vi "PLL Final.vi"() -> ()   [LabVIEW 2009]
uses:
  <vilib>/Instr/_visa.llb/VISA Configure Serial Port (Instr).vi
panel:
  in  "SDR RS232 CONTROLLER 2":T1(tab)
  in  "Stop":bool
  in  "Verzend":bool
  in  "BAND SELECTOR":dbl(ring)
  out "Ingesteld?":bool
  in  "VISA resource name":refnum<visa-resource-name>="COM1"
  in  "data bits":u16=8 min=5 max=8 step=1
  in  "baud rate":u32=9600
  out "Ingestelde frequenties":dbl(graph)
  # "PRIORITY SETTINGS"
  # "Software Defined Radio Controller SDRC3264 English\n\n  Copyright (C) 2010-2011 , All rights reserved.\n  \n\n  Software Defined Radio is being developed by:\n                - Jeroen Croes\n                - Elisa Staelen\n                - Tom Grenson\n\n\n\n  This software is packaged using NI LabView by National Instruments\n  (www.http://www.ni.com/labview/)."
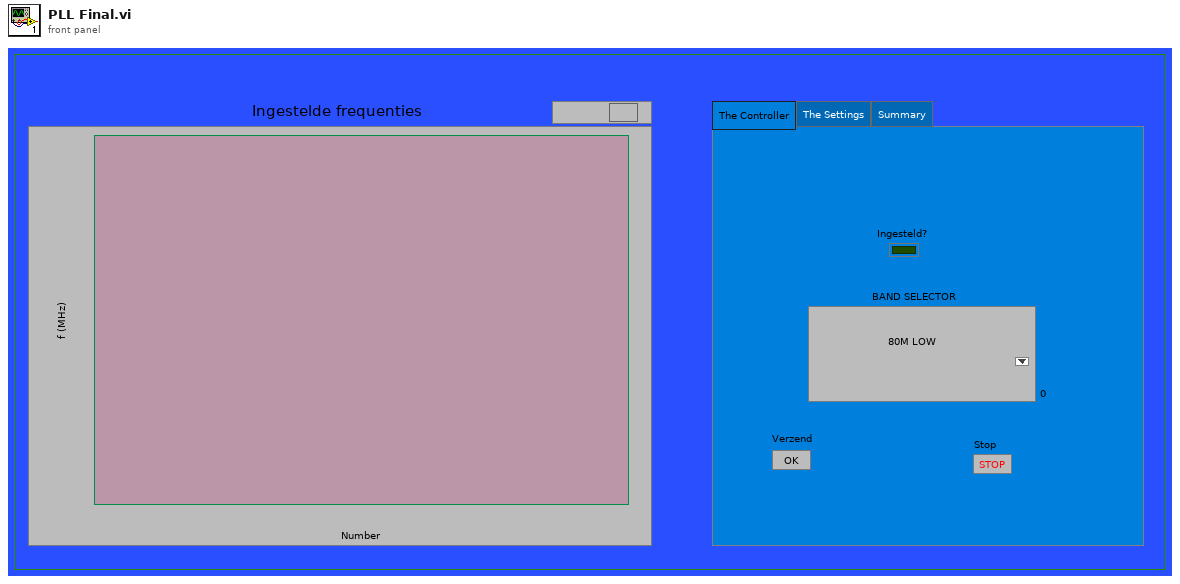
[diagram p1: front panel]
types:
  T1 = enum32{"The Controller", "The Settings", "Summary"}
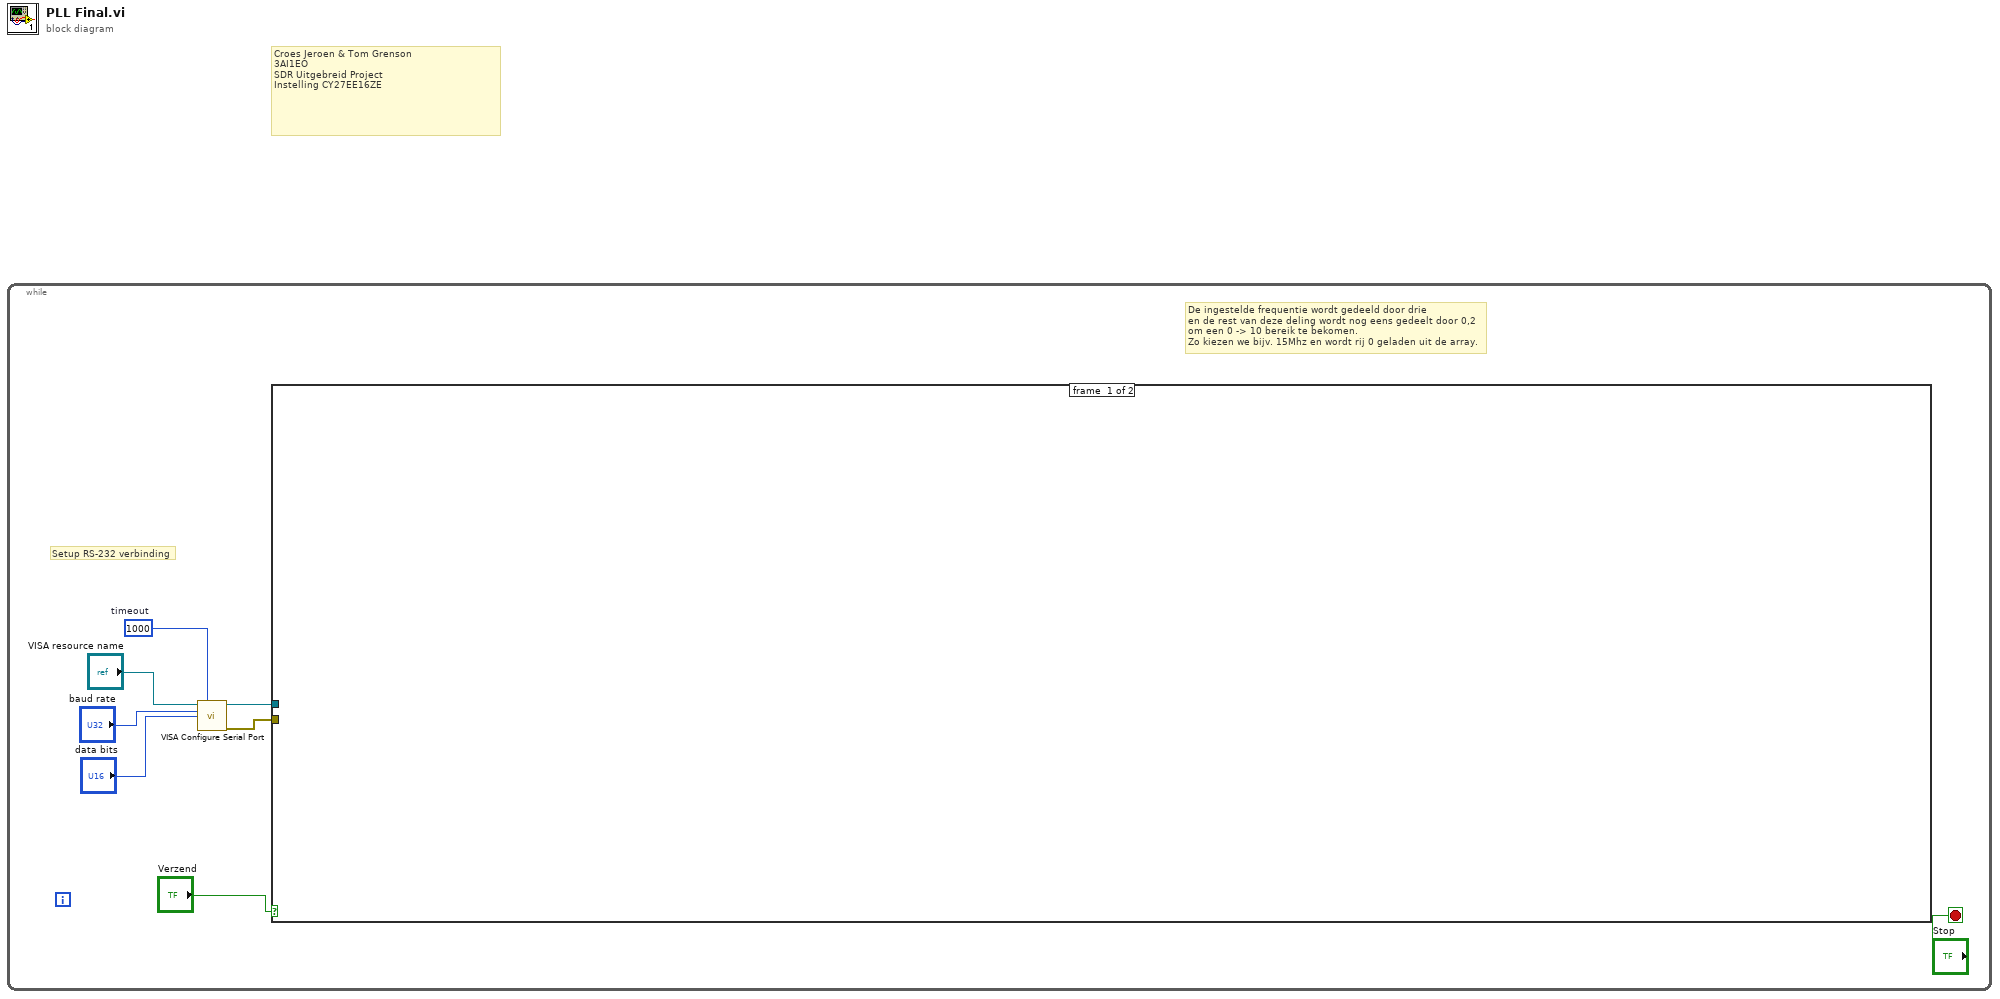
[diagram p0: block diagram]
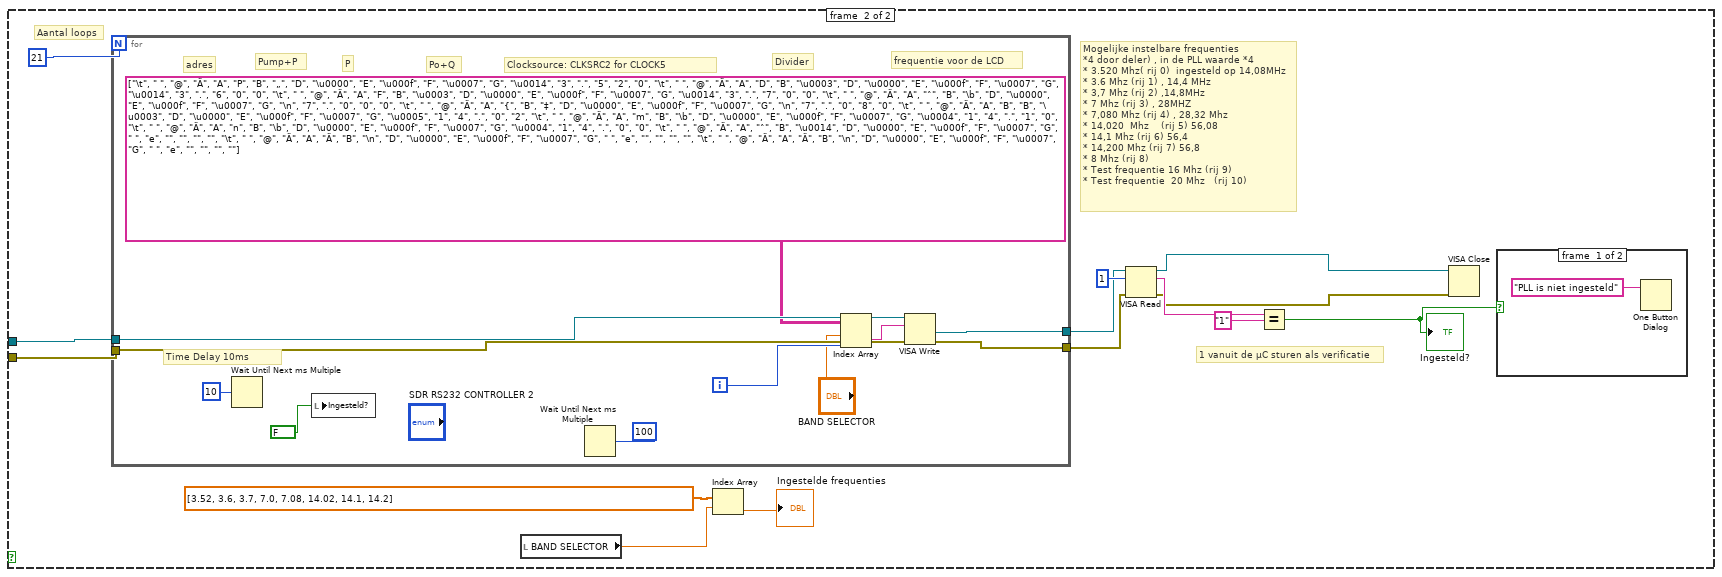
[diagram p2: hidden frame]
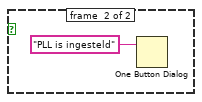
[diagram p3: hidden frame]
diagram:
  # "Croes Jeroen & Tom Grenson\n3AI1EO\nSDR Uitgebreid Project\nInstelling CY27EE16ZE"
  n1 = while {
    stop <- "Stop" stop-if-true
    w8 = u32 1000  # timeout
    # "De ingestelde frequentie wordt gedeeld door drie\nen de rest van deze deling wordt nog eens gedeelt door 0,2\nom een 0 -> 10 bereik te bekomen.\nZo kiezen we bijv. 15Mhz en wordt rij 0 geladen uit de array."
    # "Setup RS-232 verbinding"
    n2 = call-poly "VISA Configure Serial Port"("VISA resource name"="VISA resource name", "timeout (10sec)"=w8, "baud rate (9600)"="baud rate", "data bits (8)"="data bits") -> ("VISA resource name out"=w7:refnum<visa-resource-name>, "error out"=w3:errorcluster)  [unwired: 3 in, 7 out]
    n3 = case shown="True" "Verzend" {
      tunnel: w7 -> [_ w21]
      tunnel: w3 -> [_ w9]
      frame #0 {
      }
      frame #1 {
        # "Aantal loops"
        # "1 vanuit de µC sturen als verificatie"
        # "Mogelijke instelbare frequenties \n*4 door deler) , in de PLL waarde *4\n* 3.520 Mhz( rij 0)  ingesteld op 14,08MHz\n* 3.6 Mhz (rij 1) , 14,4 MHz\n* 3,7 Mhz (rij 2) ,14,8MHz\n* 7 Mhz (rij 3) , 28MHZ\n* 7,080 Mhz (rij 4) , 28,32 Mhz \n* 14,020  Mhz    (rij 5) 56,08\n* 14,1 Mhz (rij 6) 56,4\n* 14,200 Mhz (rij 7) 56,8\n* 8 Mhz (rij 8)\n* Test frequentie 16 Mhz (rij 9)\n* Test frequentie  20 Mhz   (rij 10)"
        n4 = for {
          N: 21 -> [_]
          tunnel: w21 -> [w35]
          tunnel: w9 -> [w34]
          tunnel: [w32] -> w16
          tunnel: [w28] -> w17
          i -> [w29]
          # "Divider"
          # "Clocksource: CLKSRC2 for CLOCK5"
          # "adres"
          # "P"
          # "Pump+P"
          # "Po+Q"
          # "frequentie voor de LCD"
          # "Time Delay 10ms"
          n5 = Wait Until Next ms Multiple(millisecond multiple=u32 10) -> ()  [unwired: 1 out]
          n6 = local write "Ingesteld?"(FALSE) -> ()
          n7 = Wait Until Next ms Multiple(millisecond multiple=u32 100) -> ()  [unwired: 1 out]
          n8 = Index Array(array=string[][] [["\t", " ", "@", "Ä", "A", "P", "B", "„", "D", "\u0000", "E", "\u000f", "F", "\u0007", "G", "\u0014", "3", ".", "5", "2", "0"], ["\t", " ", "@", "Ä", "A", "D", "B", "\u0003", "D", "\u0000", "E", "\u000f", "F", "\u0007", "G", "\u0014", "3", ".", "6", "0", "0"], ["\t", " ", "@", "Ä", "A", "F", "B", "\u0003", "D", "\u0000", "E", "\u000f", "F", "\u0007", "G", "\u0014", "3", ".", "7", "0", "0"], ["\t", " ", "@", "Ä", "A", "ˆ", "B", "\b", "D", "\u0000", "E", "\u000f", "F", "\u0007", "G", "\n", "7", ".", "0", "0", "0"], ["\t", " ", "@", "Ä", "A", "{", "B", "‡", "D", "\u0000", "E", "\u000f", "F", "\u0007", "G", "\n", "7", ".", "0", "8", "0"], ["\t", " ", "@", "Ä", "A", "B", "B", "\u0003", "D", "\u0000", "E", "\u000f", "F", "\u0007", "G", "\u0005", "1", "4", ".", "0", "2"], ["\t", " ", "@", "Ä", "A", "m", "B", "\b", "D", "\u0000", "E", "\u000f", "F", "\u0007", "G", "\u0004", "1", "4", ".", "1", "0"], ["\t", " ", "@", "Ä", "A", "n", "B", "\b", "D", "\u0000", "E", "\u000f", "F", "\u0007", "G", "\u0004", "1", "4", ".", "0", "0"], ["\t", " ", "@", "Ä", "A", "ˆ", "B", "\u0014", "D", "\u0000", "E", "\u000f", "F", "\u0007", "G", " ", "e", "", "", "", ""], ["\t", " ", "@", "Ä", "A", "Ä", "B", "\n", "D", "\u0000", "E", "\u000f", "F", "\u0007", "G", " ", "e", "", "", "", ""], ["\t", " ", "@", "Ä", "A", "Ä", "B", "\n", "D", "\u0000", "E", "\u000f", "F", "\u0007", "G", " ", "e", "", "", "", ""]], index (row)="BAND SELECTOR", index (col)=w29) -> (element=w31:string)
          n9 = VISA Write(VISA resource name=w35, write buffer=w31, error in (no error)=w34) -> (VISA resource name out=w32:refnum<visa-resource-name>, error out=w28:errorcluster)  [unwired: 1 out]
        }
        n10 = local read "BAND SELECTOR"() -> (w10:dbl)
        n11 = Index Array(array=dbl[] [3.52, 3.6, 3.7, 7.0, 7.08, 14.02, 14.1, 14.2], index=w10) -> (element=→"Ingestelde frequenties":dbl)
        n12 = VISA Read(VISA resource name=w16, byte count=u32 1, error in (no error)=w17) -> (VISA resource name out=w15:refnum<visa-resource-name>, read buffer=w19:string, error out=w14:errorcluster)  [unwired: 1 out]
        n13 = Equal?(x=w19, y="1") -> (x = y?=w13:bool)
        "Ingesteld?" <- w13
        n14 = VISA Close(VISA resource name=w15, error in (no error)=w14) -> ()  [unwired: 1 out]
        n15 = case shown="False" w13 {
          frame #0 {
            n16 = One Button Dialog(message="PLL is niet ingesteld") -> ()  [unwired: 1 in, 1 out]
          }
          frame #1 {
            n17 = One Button Dialog(message="PLL is ingesteld") -> ()  [unwired: 1 in, 1 out]
          }
        }
      }
    }
  }
